vi "Update Relay State.vi"(7 "position":T1=10 items=["Open"=10, "Closed"=11], 8 "error in (no error)":errorcluster, 10 "relay string":string, 11 "Route Manager in":refnum<class "Route Manager.lvclass">) -> (0 "error out":errorcluster, 3 "Route Manager out":refnum<class "Route Manager.lvclass">)   [LabVIEW 2015, in "Route Manager.lvclass"]
uses:
  Route Manager.lvclass
  Position.ctl
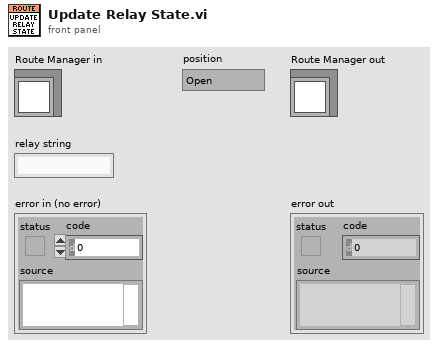
[diagram p1: front panel]
types:
  T1 = typedef "Route Manager.lvclass/Position.ctl" = i32
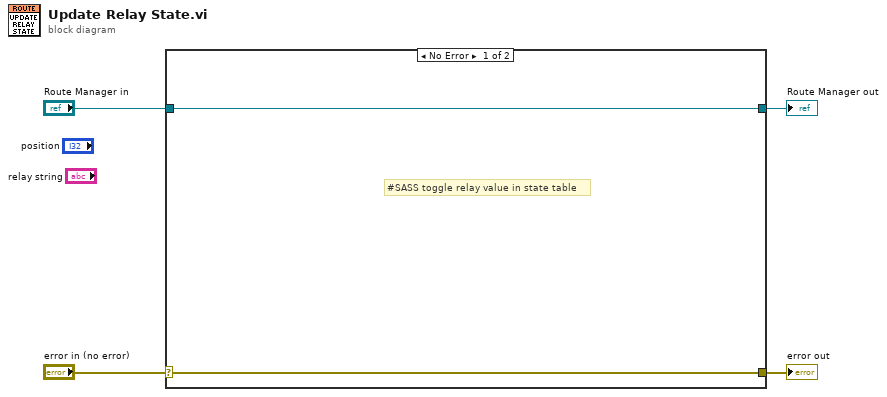
[diagram p0: block diagram]
diagram:
  n1 = case shown="No Error" "error in (no error)" {
    selector: "error in (no error)" -> [w6 w8]
    tunnel: [w6 w8] -> w3
    tunnel: [w5 w7] -> w1
    tunnel: "Route Manager in" -> [w5 w7]
    frame No Error {
      # "#SASS toggle relay value in state table"
    }
    frame Error {
      # "Error occured, so don't update state"
    }
  }
  "error out" <- w3
  "Route Manager out" <- w1
